vi "Test_camera.vi"() -> ()   [LabVIEW 2019]
uses:
  controls/Data.ctl
  <vilib>/userdefined/High Color/IMAQdx.ctl
  <vilib>/vision/Image Controls.llb/IMAQ Image.ctl
  controls/State.ctl
  <vilib>/Platform/TimedLoop/XDataNode/timing_clust.ctl
  <vilib>/Platform/TimedLoop/XDataNode/nitl_modes.ctl
  <vilib>/Platform/TimedLoop/XDataNode/wakeup.ctl
  <extravilib>/ChannelInstances/Tag-t'Data.ctl'/Read With Abort.vi
  <extravilib>/ChannelInstances/Stream-t'IMAQ Image.ctl'/Write With Abort.vi
  <extravilib>/ChannelInstances/Tag-bool/Read With Abort.vi
  <extravilib>/ChannelInstances/Tag-bool/Write With Abort.vi
  <extravilib>/ChannelInstances/Tag-t'Data.ctl'/Write With Abort.vi
  <extravilib>/ChannelInstances/Stream-t'IMAQ Image.ctl'/Endpoint.vi
  <extravilib>/ChannelInstances/Stream-t'IMAQ Image.ctl'/Instantiate.vi
  <extravilib>/ChannelInstances/Tag-bool/Instantiate.vi
  <extravilib>/ChannelInstances/Tag-t'Data.ctl'/Instantiate.vi
  <extravilib>/ChannelInstances/Tag-bool/Endpoint.vi
  <extravilib>/ChannelInstances/Tag-t'Data.ctl'/Endpoint.vi
  <extravilib>/ChannelInstances/Tag-t'Data.ctl'/EndpointRead.vi
  <extravilib>/ChannelInstances/Stream-t'IMAQ Image.ctl'/)Channel.vi
  <resource>/ChannelSupport/_ChannelSupport/WaitIfNeeded.vi
  <extravilib>/ChannelInstances/Tag-bool/EndpointRead.vi
  <vilib>/platform/TimedLoop/XDataNode/XDataNode.xnode
  <vilib>/Platform/TimedLoop/XDataNode/XDNodeRunTimeDep.lvlib
  <extravilib>/ChannelInstances/Tag-bool.lvlib
  <extravilib>/ChannelInstances/Tag-t'Data.ctl'.lvlib
  <extravilib>/ChannelInstances/Stream-t'IMAQ Image.ctl'.lvlib
panel:
  out "error out":errorcluster
  out "Cam2":T1(plugin-control)
  in  "Exposure Time":dbl=3000.0
  in  "Stop":bool
  out "Cam1":T1(plugin-control)
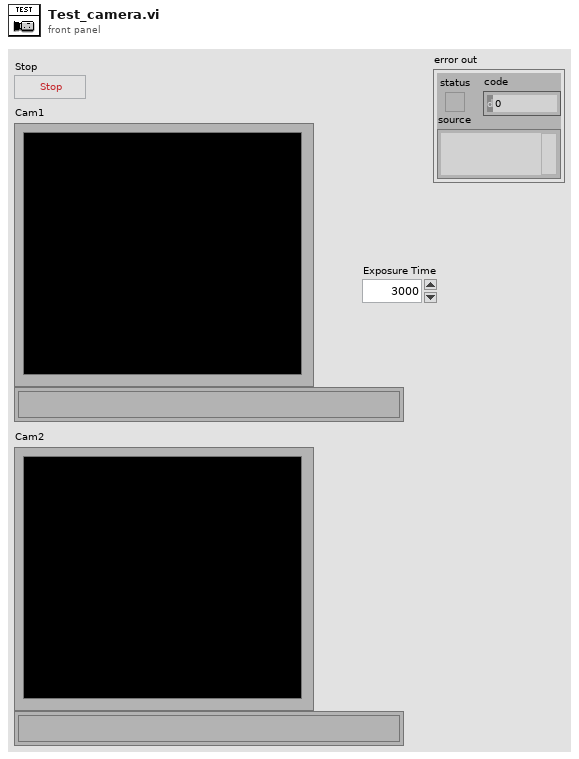
[diagram p1: front panel]
types:
  T1 = typedef "IMAQ Image.ctl" = refnum<image>
  T2 = typedef "State.ctl" = enum16{"Initialize", "Wait for Event", "Manual Cycle", "Position", "Manual Extend", "Manual Retract", "Initialize Pump", "Pump Top", "Pump Bottom", "Pump Terminate", "Pump Cycle", "Connect Systems", "Start Image Capture", "Stop Image Capture", "Calibration Pictures", "Empty and Refill", "Change Light Intensity", "Reconnect", "Exit"}
  T3 = typedef "Data.ctl" = cluster{"L16 Linear Actuator":refnum<visa-resource-name>, "XE 1000 Pump":refnum<visa-resource-name>, "Camera1":T4, "Camera2":T4, "Camera1_IMG":T1, "Camera2_IMG":T1, "Img_Capt":bool, "Actuator":bool, "Pump":bool, "Cam 1":bool, "Cam 2":bool, "Empty_Refill":bool, "Crop":bool, "Period":i64, "Light intensity":i32, "Exposure Time":dbl, "Sample Name":string, "Operator":string, "Calibration 1":path, "Calibration 2":path, "Save frequency":i32, "Timeout Sample":i32, "Sample Frequency":i32, "Notes/Description":string}
  T4 = typedef "IMAQdx.ctl" = refnum<k21>
  T5 = typedef "XDNodeRunTimeDep.lvlib/timing_clust.ctl" = cluster{"Expected End [f-1]":u64, "Actual End [f-1]":u64, "Finished Late? [f-1]":bool, "Expected End [i-1]":u64, "Actual End [i-1]":u64, "Finished Late? [i-1]":bool, "Expected Start [i]":u64, "Actual Start [i]":u64, "Expected Start [f]":u64, "Actual Start [f]":u64, "Source Name":string, "Structure Name":string, "Period":i64, "Deadline":i64, "Offset":i64, "Start":i64, "Priority":i32, "Timeout":i32, "Mode":T6, "Wakeup Reason":T7, "Error":errorcluster, "Source Type":string, "Secondary Source Type":string, "Global End Time":u64, "Global Start Time":u64, "Frame Duration":u64, "Iteration Duration":u64, "Assigned CPU":i32, "I/O Scan Engine Mode":u32}
  T6 = typedef "XDNodeRunTimeDep.lvlib/nitl_modes.ctl" = enum32{"No Change", "Process missed periods, maintain original phase", "Discard missed periods, maintain original phase", "Process missed periods, ignore original phase", "Discard missed periods, ignore original phase"}
  T7 = typedef "XDNodeRunTimeDep.lvlib/wakeup.ctl" = enum32{"Normal", "Aborted", "Asynchronous wakeup", "Timing source error", "Timed loop error", "Timeout"}
  T8 = typedef "Tag-bool.lvlib/))Channel.ctl" = refnum<queue>
  T9 = typedef "Tag-t'Data.ctl'.lvlib/))Channel.ctl" = refnum<queue>
  T10 = typedef "Stream-t'IMAQ Image.ctl'.lvlib/)Channel.ctl" = refnum<queue>
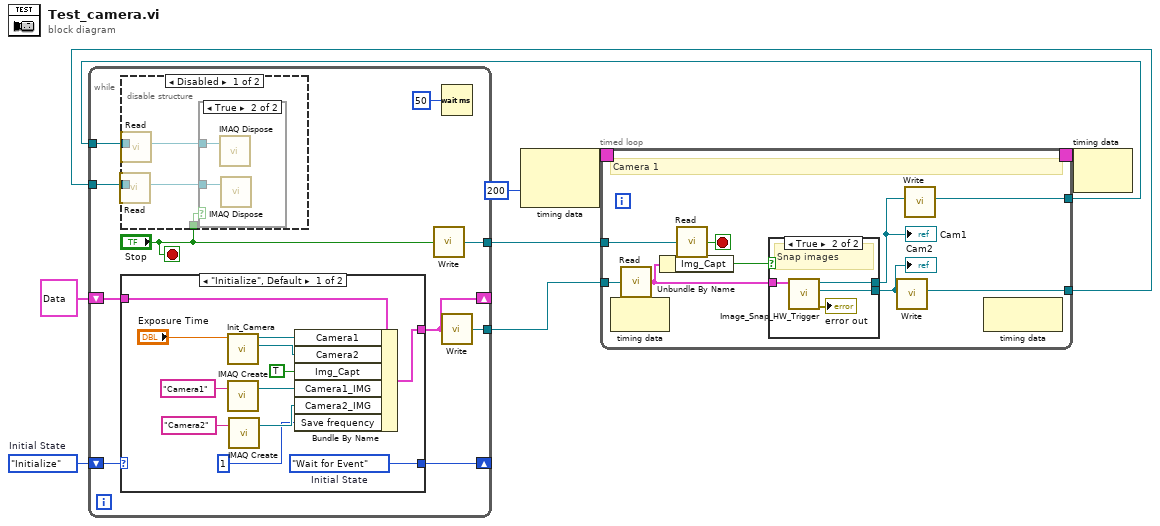
[diagram p0: block diagram]
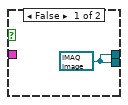
[diagram p2: hidden frame]
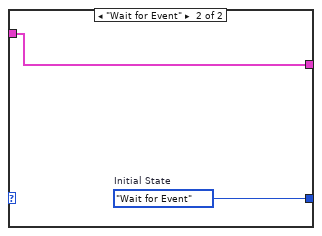
[diagram p5: hidden frame]
diagram:
  w7 = State."Initialize"  # Initial State
  n1 = node-c288(i64 200 ("Period")) -> (w4:T5)  [unwired: 1 in]
  n2 = while {
    tunnel: [w19] -> w6
    tunnel: [w18] -> w5
    tunnel: w9 -> [w17]
    shift-right: [w15] -> _
    shift-left: T3 {"L16 Linear Actuator"="", "XE 1000 Pump"="", "Camera1"="", "Camera2"="", "Camera1_IMG"=refnum, "Camera2_IMG"=refnum, "Img_Capt"=FALSE, "Actuator"=FALSE, "Pump"=FALSE, "Cam 1"=FALSE, "Cam 2"=FALSE, "Empty_Refill"=FALSE, "Crop"=FALSE, "Period"=0, "Light intensity"=100, "Exposure Time"=1000.0, "Sample Name"="Test Sample", "Operator"="MRJ", "Calibration 1"=path "C:/Users/au540322/Desktop/IHS_Project/images/Debris/Debris_0/Debris_0_2019_06_01-23-32-49-686.PNG", "Calibration 2"=path "C:/Users/au540322/Desktop/IHS_Project/images/Debris/Debris_0/Debris_0_2019_06_01-23-32-49-686.PNG", "Save frequency"=1, "Timeout Sample"=200, "Sample Frequency"=200, "Notes/Description"=""} ("Data") -> [w16]
    shift-right: [w12] -> _
    shift-left: w7 -> [w14]
    tunnel: w1 -> [w10]
    stop <- "Stop" stop-if-true
    n3 = case shown="\"Initialize\", Default" w14 {
      tunnel: [w30 w39] -> w15
      tunnel: w16 -> [w36 w39]
      tunnel: [w35 w40] -> w12
      frame "Initialize", Default {
        w35 = State."Wait for Event"  # Initial State
        n4 = call "Init_Camera.vi"("Exposure Time"="Exposure Time") -> ("Camera2"=w37:T4, "Camera1"=w38:T4)  [unwired: 7 in, 2 out]
        n5 = call "IMAQ Create"("Image Name"="Camera1") -> ("New Image"=w31:T1)  [unwired: 4 in, 1 out]
        n6 = call "IMAQ Create"("Image Name"="Camera2") -> ("New Image"=w28:T1)  [unwired: 4 in, 1 out]
        n7 = Bundle By Name(cluster=w36, "Camera1"=w38, "Camera2"=w37, "Img_Capt"=TRUE, "Camera1_IMG"=w31, "Camera2_IMG"=w28, "Save frequency"=1) -> (w30:T3)
      }
      frame "Wait for Event" {
        w40 = State."Wait for Event"  # Initial State
      }
    }
    n8 = disable-structure shown="Disabled" {
      disable-tunnel: w17 -> [w24 _]
      disable-tunnel: "Stop" -> [w23 _]
      disable-tunnel: w10 -> [w21 _]
      frame Disabled {
        n9 = call <extravilib>:"Read.vi"("channel"=w21) -> ("element"=w22:T1)  [unwired: 6 in, 4 out]
        n10 = call <extravilib>:"Read.vi"("channel"=w24) -> ("element"=w20:T1)  [unwired: 6 in, 4 out]
        n11 = case shown="True" w23 {
          tunnel: w20 -> [_ w26]
          tunnel: w22 -> [_ w25]
          frame False {
          }
          frame True {
            n12 = call "IMAQ Dispose"("Image"=w26) -> ()  [unwired: 5 in, 1 out]
            n13 = call "IMAQ Dispose"("Image"=w25) -> ()  [unwired: 5 in, 1 out]
          }
        }
      }
      frame Enabled {
      }
    }
    n14 = call <extravilib>:"Write.vi"("element"="Stop") -> ("channel"=w18:T8)  [unwired: 1 out]
    n15 = Wait (ms)(milliseconds to wait=u32 50) -> ()  [unwired: 1 out]
    n16 = call <extravilib>:"Write.vi"("element"=w15) -> ("channel"=w19:T9)  [unwired: 1 out]
  }
  n17 = timed-loop {
    timing: w4 -> [_]
    timing-out: [_] -> w3
    tunnel: w5 -> [w49]
    tunnel: w6 -> [w48]
    tunnel: [w45] -> w9
    tunnel: [w42] -> w1
    stop <- w41 stop-if-true
    # "Camera 1"
    n18 = node-c288() -> ()  [unwired: 1 in, 1 out]
    n19 = call <extravilib>:"Read.vi"("channel"=w48) -> ("element"=w46:T3)  [unwired: 1 in, 1 out]
    n20 = Unbundle By Name(w46) -> ("Img_Capt"=w47:bool)
    n21 = call <extravilib>:"Read.vi"("channel"=w49) -> ("element"=w41:bool)  [unwired: 1 in, 1 out]
    n22 = case shown="True" w47 {
      tunnel: w46 -> [_ w54]
      tunnel: [w50 w53] -> w44
      tunnel: [w50 w52] -> w43
      frame False {
        w50 = T1 refnum ("Image Out")
      }
      frame True {
        # "Snap images"
        n23 = call "Image_Snap_HW_Trigger.vi"("input cluster"=w54) -> ("error out"=→"error out":errorcluster, "Image2"=w52:T1, "Image1"=w53:T1)  [unwired: 8 in]
      }
    }
    "Cam1" <- w44
    "Cam2" <- w43
    n24 = call <extravilib>:"Write.vi"("element"=w43) -> ("channel"=w42:T10)  [unwired: 8 in, 2 out]
    n25 = call <extravilib>:"Write.vi"("element"=w44) -> ("channel"=w45:T10)  [unwired: 8 in, 2 out]
    n26 = node-c288() -> ()  [unwired: 1 in, 1 out]
  }
  n27 = node-c288(w3) -> ()  [unwired: 1 out]
